vi "thresholdCalculator.vi"() -> ()   [LabVIEW 2012]
panel:
  in  "std deviations":dbl=4.0
  out "Dark Level out":dbl
  out "Bright Level out":dbl
  out "Threshold":dbl
  out "output exposure time":dbl
  in  "Input Exposure Time":dbl
  in  "Bright Level":dbl
  in  "Dark Level":dbl
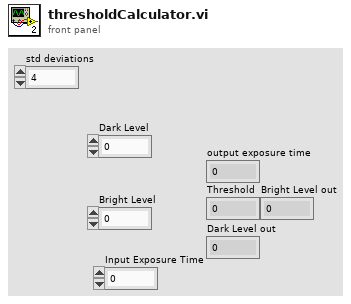
[diagram p1: front panel]
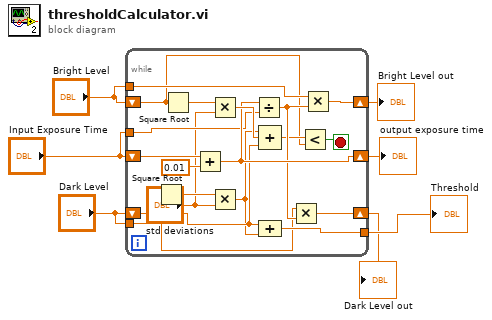
[diagram p0: block diagram]
diagram:
  n1 = while {
    tunnel: "Input Exposure Time" -> [w12]
    shift-right: [w21] -> w6
    shift-left: "Input Exposure Time" -> [w23]
    shift-right: [w18] -> w4
    shift-left: "Bright Level" -> [w9]
    shift-right: [w19] -> w3
    shift-left: "Dark Level" -> [w17]
    tunnel: [w15] -> w5
    tunnel: "Dark Level" -> [w11]
    tunnel: "Bright Level" -> [w10]
    stop <- w13 stop-if-true
    n2 = Square Root(x=w17) -> (sqrt(x)=w26:dbl)
    n3 = Square Root(x=w9) -> (sqrt(x)=w25:dbl)
    n4 = Add(x=w23, y=0.01) -> (x+y=w21:dbl)
    n5 = Multiply(x=w25, y="std deviations") -> (x*y=w24:dbl)
    n6 = Multiply(x=w26, y="std deviations") -> (x*y=w16:dbl)
    n7 = Divide(x=w21, y=w12) -> (x/y=w20:dbl)
    n8 = Compound Arithmetic op=ADD(w16, w24, w17) -> (w14:dbl)
    n9 = Compound Arithmetic op=ADD(w17, w16) -> (w15:dbl)
    n10 = Multiply(x=w11, y=w20) -> (x*y=w19:dbl)
    n11 = Less?(x=w14, y=w9) -> (x < y?=w13:bool)
    n12 = Multiply(x=w10, y=w20) -> (x*y=w18:dbl)
  }
  "output exposure time" <- w6
  "Threshold" <- w5
  "Bright Level out" <- w4
  "Dark Level out" <- w3
